vi "Notifier Test.vi"() -> ()   [LabVIEW 2020]
panel:
  out "sent":i32
  out "received":i32
  in  "stop":bool
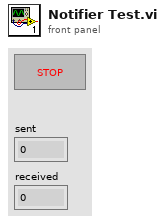
[diagram p1: front panel]
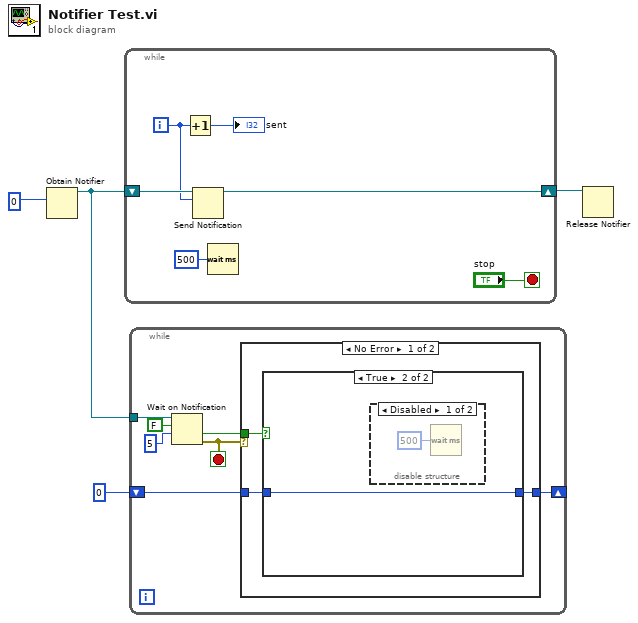
[diagram p0: block diagram]
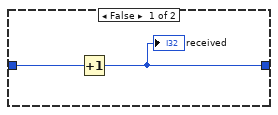
[diagram p2: hidden frame]
diagram:
  n1 = Obtain Notifier(notification data type=0) -> (notifier out=w3:refnum<notifier>)  [unwired: 3 in, 2 out]
  n2 = while {
    shift-right: [w7] -> w4
    shift-left: w3 -> [w8]
    i -> [w5]
    stop <- "stop" stop-if-true
    n3 = Increment(x=w5) -> (x+1=→"sent":i32)
    n4 = Send Notification(notification=w5, notifier=w8) -> (notifier out=w7:refnum<notifier>)  [unwired: 1 in, 1 out]
    n5 = Wait (ms)(milliseconds to wait=u32 500) -> ()  [unwired: 1 out]
  }
  n6 = while {
    tunnel: w3 -> [w17]
    shift-right: [w13] -> _
    shift-left: 0 -> [w14]
    stop <- w15 stop-if-true
    n7 = Wait on Notification(notifier=w17, ignore previous (F)=FALSE, timeout in ms (-1)=5) -> (timed out?=w16:bool, error out=w15:errorcluster)  [unwired: 1 in, 2 out]
    n8 = case shown="No Error" w15 {
      tunnel: w16 -> [w20 _]
      tunnel: w14 -> [w19 w25]
      tunnel: [w18 w25] -> w13
      frame No Error {
        n9 = case shown="True" w20 {
          tunnel: w19 -> [w22 w23]
          tunnel: [w21 w23] -> w18
          frame False {
            n10 = Increment(x=w22) -> (x+1=w21:i32)
            "received" <- w21
          }
          frame True {
            n11 = disable-structure shown="Disabled" {
              frame Disabled {
                n12 = Wait (ms)(milliseconds to wait=u32 500) -> ()  [unwired: 1 out]
              }
              frame Enabled {
              }
            }
          }
        }
      }
      frame Error {
      }
    }
  }
  n13 = Release Notifier(notifier=w4) -> ()  [unwired: 2 in, 3 out]
